vi "dfd_NStage Interpolation Rational Design.vi"(6 "fs in":dbl, 8 "error in":errorcluster, 9 "ripple specs":T2, 10 "freq specs [Hz]":T1={"fpass"=45.0, "fstop"=52.0}, 11 "manual factorization in":T3[](array[typedef])) -> (0 "error out":errorcluster, 3 "multirate filter out":T4[](array[typedef]) {"mSRate_QSettings"."source" items=["Coef a/k"=0, "Coef b/v"=7, "Input"=1, "Output"=2, "Multiplicand"=3, "Product"=4, "Sum"=5, "Delay"=6, "Gain"=8]})   [LabVIEW 2017, in "NI_DigFilterLicensed.lvlib"]
uses:
  <vilib>/addons/Digital Filter Design/NI_DigFilterLicensed.lvlib
  <vilib>/addons/Digital Filter Design/_Objects.llb/DFD Filter Obj.ctl
  <vilib>/addons/Digital Filter Design/_Objects.llb/DFD Filter Coef.ctl
  <vilib>/addons/Digital Filter Design/_Objects.llb/DFD Filter Structure Type Selector.ctl
  <vilib>/addons/Digital Filter Design/_Objects.llb/dfd_Internal Quantization Settings.ctl
  <vilib>/addons/Digital Filter Design/_Objects.llb/dfd_Internal Quantization Srcs.ctl
  <vilib>/addons/Digital Filter Design/_Objects.llb/DFD Coef Norm Type.ctl
  <vilib>/addons/Digital Filter Design/_Objects.llb/DFD Multirate Rational Factor.ctl
  <vilib>/addons/Digital Filter Design/_Objects.llb/DFD Filter Ripple Specification (Design).ctl
  <vilib>/addons/Digital Filter Design/_Objects.llb/DFD Multirate Filter Specification (Design).ctl
  <vilib>/addons/Digital Filter Design/_Objects.llb/DFD Filter Frequence Specification (Design).ctl
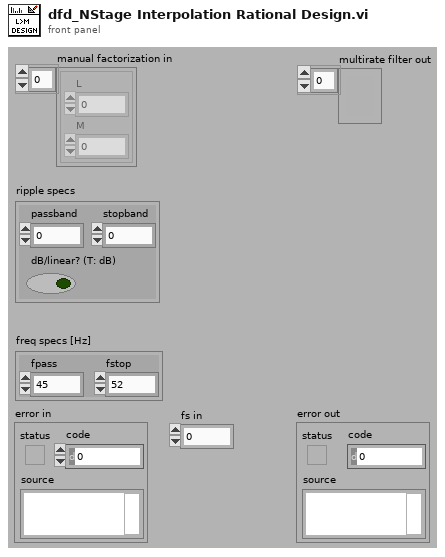
[diagram p1: front panel]
types:
  T1 = typedef "NI_DigFilterLicensed.lvlib/DFD Multirate Filter Specification (Design).ctl" = cluster{"fpass":dbl, "fstop":dbl}
  T2 = typedef "NI_DigFilterLicensed.lvlib/DFD Filter Ripple Specification (Design).ctl" = cluster{"passband":dbl, "stopband":dbl, "dB/linear? (T: dB)":bool}
  T3 = typedef "NI_DigFilterLicensed.lvlib/DFD Multirate Rational Factor.ctl" = cluster{"L":i32, "M":i32}
  T4 = typedef "NI_DigFilterLicensed.lvlib/DFD Filter Obj.ctl" = cluster{"mSRate_Fs":dbl, "mSRate_Version":string, "mSRate_Comments":string, "mSRate_OrgCoef":T5, "mSRate_CurCoef":T5, "mSRate_Quantized?":bool, "mSRate_QCoef":T5, "mSRate_QSettings":T7[], "mSRate_Order":i32, "mSRate_Scaling":cluster{"mSRate_ScaleByPowerOf2?":bool, "mSRate_ScaleType":T9}}
  T5 = typedef "NI_DigFilterLicensed.lvlib/DFD Filter Coef.ctl" = cluster{"type":T6, "gain":dbl, "coef a (k)":dbl[], "coef b (v)":dbl[]}
  T6 = typedef "NI_DigFilterLicensed.lvlib/DFD Filter Structure Type Selector.ctl" = enum16{"Undefined", "FIR Direct Form", "FIR Direct Form Transposed", "FIR Symmetric", "FIR Antisymmetric", "IIR Direct Form I", "IIR Direct Form I Transposed", "IIR Direct Form II", "IIR Direct Form II Transposed", "IIR Cascaded Second Order Sections Form I", "IIR Cascaded Second Order Sections Form I Transposed", "IIR Cascaded Second Order Sections Form II", "IIR Cascaded Second Order Sections Form II Transposed", "Lattice Allpass (basic sections)", "Lattice Allpass (one multiplier sections)", "Lattice Allpass (normalized sections)", "Lattice AR (basic sections)", "Lattice AR (one multiplier sections)", "Lattice AR (normalized sections)", "Lattice MA (minimum phase)", "Lattice MA (maximum phase)", "Lattice ARMA (basic sections)", "Lattice ARMA (one multiplier sections)", "Lattice ARMA (normalized sections)"}
  T7 = typedef "NI_DigFilterLicensed.lvlib/dfd_Internal Quantization Settings.ctl" = cluster{"source":T8, "wl":i16, "iwl":i16, "overflow mode":enum16{"Saturation", "Wrap"}, "rounding mode":enum16{"Nearest", "Truncation"}, "signed?":bool}
  T8 = typedef "NI_DigFilterLicensed.lvlib/dfd_Internal Quantization Srcs.ctl" = u16
  T9 = typedef "NI_DigFilterLicensed.lvlib/DFD Coef Norm Type.ctl" = enum16{"No Norm", "Time Domain 1-Norm", "Time Domain 2-Norm", "Time Domain Inf-Norm"}
  T10 = typedef "NI_DigFilterLicensed.lvlib/DFD Filter Frequence Specification (Design).ctl" = cluster{"fpass 1":dbl, "fstop 1":dbl, "fpass 2 ":dbl, "fstop 2":dbl}
  T11 = enum16{"Butterworth", "Chebyshev", "Inverse Chebyshev", "Elliptic", "Kaiser Window", "Dolph-Chebyshev Window", "Equi-Ripple FIR"}
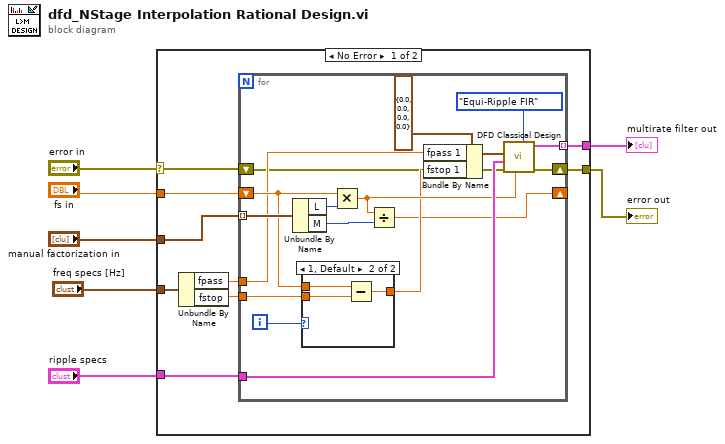
[diagram p0: block diagram]
diagram:
  n1 = case shown="No Error" "error in" {
    selector: "error in" -> [w8 w38]
    tunnel: [w16 w38] -> w2
    tunnel: "fs in" -> [w15 _]
    tunnel: [w14 _] -> w6
    tunnel: "manual factorization in" -> [w13 _]
    tunnel: "ripple specs" -> [w12 _]
    tunnel: "freq specs [Hz]" -> [w9 _]
    frame No Error {
      n2 = Unbundle By Name(w9) -> ("fpass"=w10:dbl, "fstop"=w11:dbl)
      n3 = for {
        shift-right: [w20] -> _
        shift-left: w15 -> [w27]
        tunnel: w10 -> [w25]
        tunnel: w11 -> [w32]
        tunnel: w13 -> [w30] mode=indexing
        tunnel: w12 -> [w31]
        tunnel: [w22] -> w14 mode=indexing
        shift-right: [w21] -> w16
        shift-left: w8 -> [w18]
        i -> [w33]
        n4 = Unbundle By Name(w30) -> ("L"=w19:i32, "M"=w29:i32)
        n5 = case shown="1, Default" w33 {
          tunnel: w32 -> [w34 w37]
          tunnel: [w34 w36] -> w24
          tunnel: w27 -> [_ w35]
          frame 0 {
          }
          frame 1, Default {
            n6 = Subtract(x=w35, y=w37) -> (x-y=w36:dbl)
          }
        }
        n7 = Multiply(x=w27, y=w19) -> (x*y=w28:dbl)
        n8 = Divide(x=w28, y=w29) -> (x/y=w20:dbl)
        n9 = Bundle By Name(cluster=T10 {"fpass 1"=0.0, "fstop 1"=0.0, "fpass 2 "=0.0, "fstop 2"=0.0} ("freq specs [Hz]"), "fpass 1"=w25, "fstop 1"=w24) -> (w26:T10)
        n10 = call <vilib>:"DFD Classical Design.vi"("design method"=T11."Equi-Ripple FIR", "fs [Hz]"=w28, "error in (no error)"=w18, "ripple specs"=w31, "freq specs [Hz]"=w26) -> ("error out"=w21:errorcluster, "filter out"=w22:T4)  [unwired: 1 in, 4 out]
      }
    }
    frame Error {
    }
  }
  "error out" <- w2
  "multirate filter out" <- w6
